vi "GetOSArchitecture.vi"(8 "error in (no error)":errorcluster, 11 "application in":refnum<class "application.lvclass">) -> (0 "error out":errorcluster, 2 "32bit(T)/64bit(F)":bool, 3 "application out":refnum<class "application.lvclass">)   [LabVIEW 2014, in "application.lvclass"]
uses:
  application.lvclass
panel:
  out "standard output":string
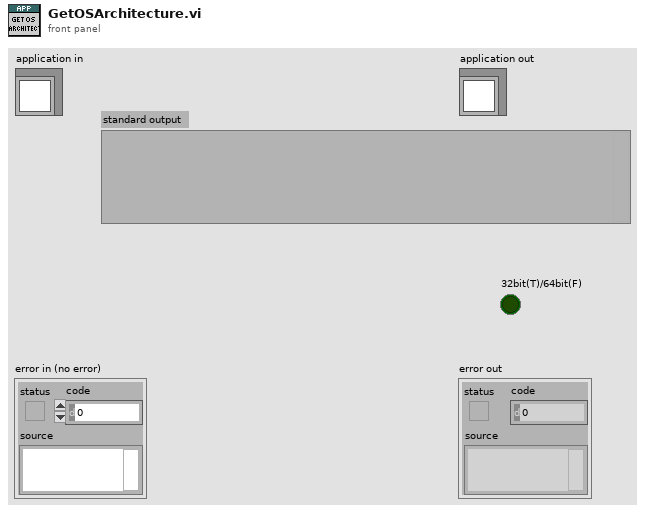
[diagram p1: front panel]
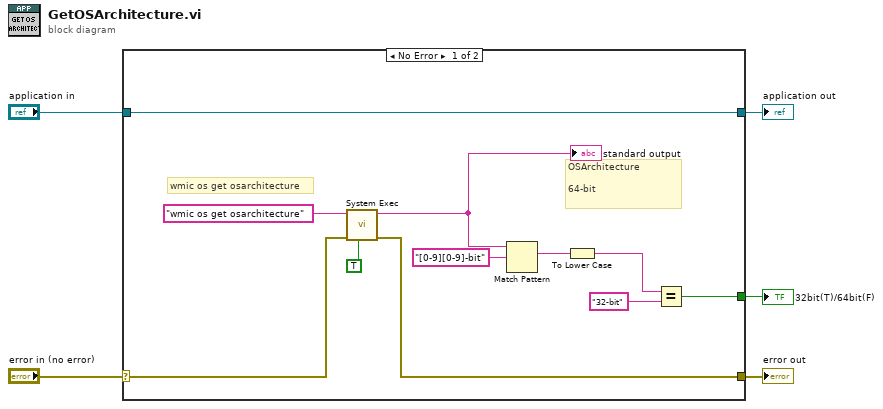
[diagram p0: block diagram]
diagram:
  n1 = case shown="No Error" "error in (no error)" {
    selector: "error in (no error)" -> [w12 w18]
    tunnel: [w11 w18] -> w4
    tunnel: [w16 w17] -> w2
    tunnel: "application in" -> [w16 w17]
    tunnel: [w8 _] -> w1
    frame No Error {
      # "OSArchitecture  \n\n64-bit"
      # "wmic os get osarchitecture"
      n2 = call <vilib>:"System Exec.vi"("run minimized? (F)"=TRUE, "error in (no error)"=w12, "command line"="wmic os get osarchitecture") -> ("error out"=w11:errorcluster, "standard output"=w14:string)  [unwired: 5 in, 2 out]
      "standard output" <- w14
      n3 = Match Pattern(string=w14, regular expression="[0-9][0-9]-bit") -> (match substring=w10:string)  [unwired: 1 in, 3 out]
      n4 = To Lower Case(string=w10) -> (all lower case string=w9:string)
      n5 = Equal?(x=w9, y="32-bit") -> (x = y?=w8:bool)
    }
    frame Error {
    }
  }
  "error out" <- w4
  "application out" <- w2
  "32bit(T)/64bit(F)" <- w1
